vi "GOOP_MouseFunctions.vi"(8 "error in (no error)":errorcluster, 9 "StabilityProblem":bool, 10 "Action(Read)":enum16{"Init", "Read", "Close"}(ring)=enum."Read") -> (0 "error out":errorcluster, 1 "button info":T1, 2 "axis info":T2)   [LabVIEW 2016]
doc: "Opens a reference to and initializes the mouse connected to the computer."
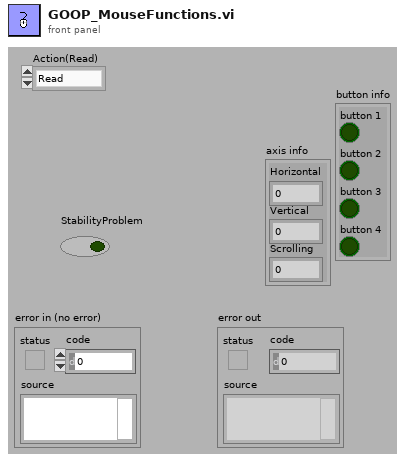
[diagram p1: front panel]
types:
  T1 = cluster{"button 1":bool, "button 2":bool, "button 3":bool, "button 4":bool}
  T2 = cluster{"Horizontal":i32, "Vertical":i32, "Scrolling":i32}
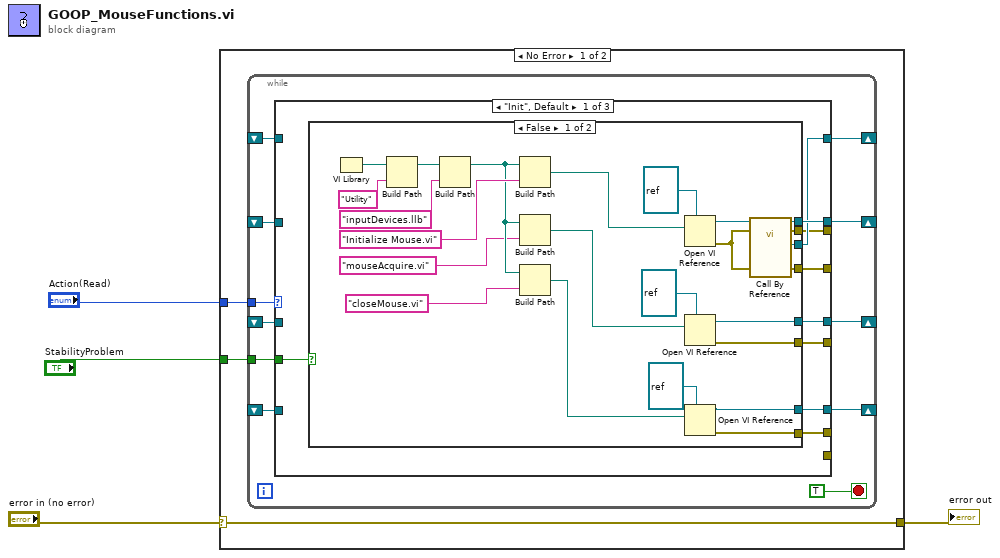
[diagram p0: block diagram]
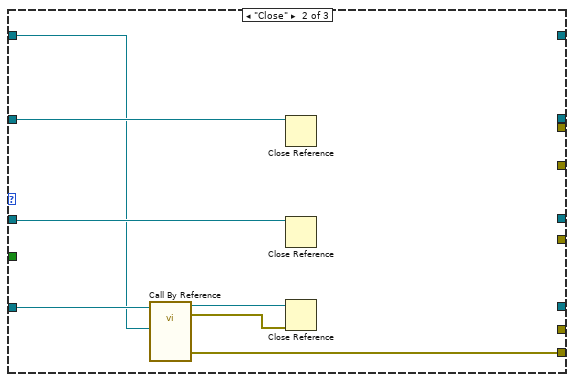
[diagram p3: hidden frame]
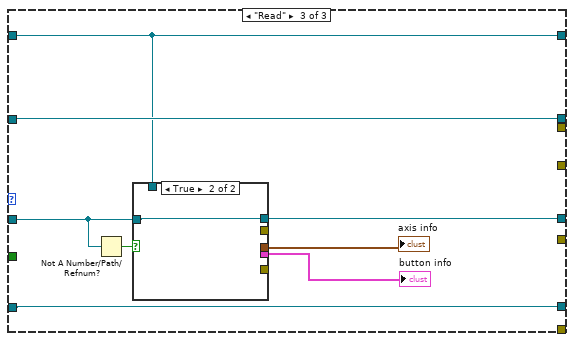
[diagram p4: hidden frame]
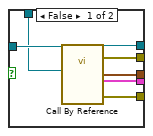
[diagram p5: hidden frame]
diagram:
  n1 = case shown="No Error" "error in (no error)" {
    selector: "error in (no error)" -> [w7 w75]
    tunnel: [w7 w75] -> w3
    tunnel: "Action(Read)" -> [w6 _]
    tunnel: "StabilityProblem" -> [w5 _]
    frame No Error {
      n2 = while {
        tunnel: w6 -> [w18]
        shift-right: [w17] -> _
        shift-left: _ -> [w16]
        shift-right: [w15] -> _
        shift-left: _ -> [w13]
        shift-right: [w14] -> _
        shift-left: _ -> [w12]
        shift-right: [w11] -> _
        shift-left: _ -> [w10]
        tunnel: w5 -> [w8]
        stop <- TRUE stop-if-true
        n3 = case shown="\"Init\", Default" w18 {
          tunnel: [w27 _ w66] -> w17
          tunnel: w16 -> [_ w54 w66]
          tunnel: [w26 _ w65] -> w15
          tunnel: [w25 _ w64] -> w14
          tunnel: w13 -> [_ w55 w61]
          tunnel: w12 -> [_ w58 w64]
          tunnel: [w24 _ w63] -> w11
          tunnel: w10 -> [_ w53 w63]
          tunnel: [w23 _ _] -> _
          tunnel: [w22 _ _] -> _
          tunnel: [w21 _ _] -> _
          tunnel: [w20 _ _] -> _
          tunnel: [_ w52 _] -> _
          tunnel: w8 -> [w19 _ _]
          frame "Init", Default {
            n4 = case shown="False" w19 {
              tunnel: [w39 _] -> w27
              tunnel: [w38 _] -> w26
              tunnel: [w37 _] -> w25
              tunnel: [w36 _] -> w24
              tunnel: [w32 _] -> w23
              tunnel: [w30 _] -> w22
              tunnel: [w29 _] -> w21
              tunnel: [w28 _] -> w20
              frame False {
                n5 = VI Library() -> (path=w51:path)
                n6 = Build Path(base path=w51, name or relative path="Utility") -> (appended path=w47:path)
                n7 = Build Path(base path=w47, name or relative path="inputDevices.llb") -> (appended path=w43:path)
                n8 = Build Path(base path=w43, name or relative path="Initialize Mouse.vi") -> (appended path=w44:path)
                n9 = Build Path(base path=w43, name or relative path="mouseAcquire.vi") -> (appended path=w35:path)
                n10 = Build Path(base path=w43, name or relative path="closeMouse.vi") -> (appended path=w34:path)
                n11 = Open VI Reference(type specifier VI Refnum (for type only)=refnum<vi> refnum, vi path=w44) -> (vi reference=w49:refnum<vi>, error out=w31:errorcluster)  [unwired: 4 in]
                n12 = Open VI Reference(type specifier VI Refnum (for type only)=refnum<vi> refnum, vi path=w35) -> (vi reference=w38:refnum<vi>, error out=w29:errorcluster)  [unwired: 4 in]
                n13 = Open VI Reference(type specifier VI Refnum (for type only)=refnum<vi> refnum, vi path=w34) -> (vi reference=w37:refnum<vi>, error out=w28:errorcluster)  [unwired: 4 in]
                n14 = call-by-ref "?"(reference=w49, error in=w31, 8:"error in (no error)"=w31) -> (reference out=w39:refnum<vi>, error out=w32:errorcluster, 0:"error out"=w30:errorcluster, "device ID"=w36:refnum<k1>)  [unwired: 9 in]
              }
              frame True {
              }
            }
          }
          frame "Close" {
            n15 = call-by-ref "?"(reference=w58, "device ID"=w53) -> (reference out=w56:refnum<vi>, error out=w57:errorcluster, 0:"error out"=w52:errorcluster)  [unwired: 10 in]
            n16 = Close Reference(reference=w54) -> ()  [unwired: 1 in, 1 out]
            n17 = Close Reference(reference=w55) -> ()  [unwired: 1 in, 1 out]
            n18 = Close Reference(reference=w56, error in (no error)=w57) -> ()  [unwired: 1 out]
          }
          frame "Read" {
            n19 = Not A Number/Path/Refnum?(number/path/refnum=w61) -> (NaN/Path/Refnum?=w62:bool)
            n20 = case shown="True" w62 {
              tunnel: w61 -> [w73 w74]
              tunnel: [w72 w74] -> w65
              tunnel: [w71 _] -> w59
              tunnel: [w70 _] -> w60
              tunnel: w63 -> [w69 _]
              tunnel: [w68 _] -> _
              tunnel: [w67 _] -> _
              frame False {
                n21 = call-by-ref "?"(reference=w73, "device ID"=w69) -> (reference out=w72:refnum<vi>, error out=w67:errorcluster, "axis info"=w70:T2, "button info"=w71:T1, 19:"error out"=w68:errorcluster)  [unwired: 16 in, 1 out]
              }
              frame True {
              }
            }
            "button info" <- w59
            "axis info" <- w60
          }
        }
      }
    }
    frame Error {
    }
  }
  "error out" <- w3
